vi "提取字符串中数字.vi"(1 "字符串":string) -> (0 "结果":string)   [LabVIEW 2014]
doc: "该模板用于创建子VI。"
panel:
  out "error out":errorcluster caption="错误输出"
  in  "error in (no error)":errorcluster caption="错误输入（无错误）"
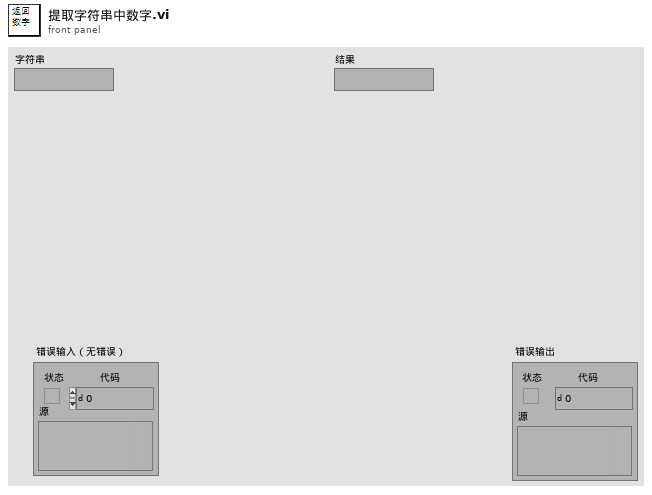
[diagram p1: front panel]
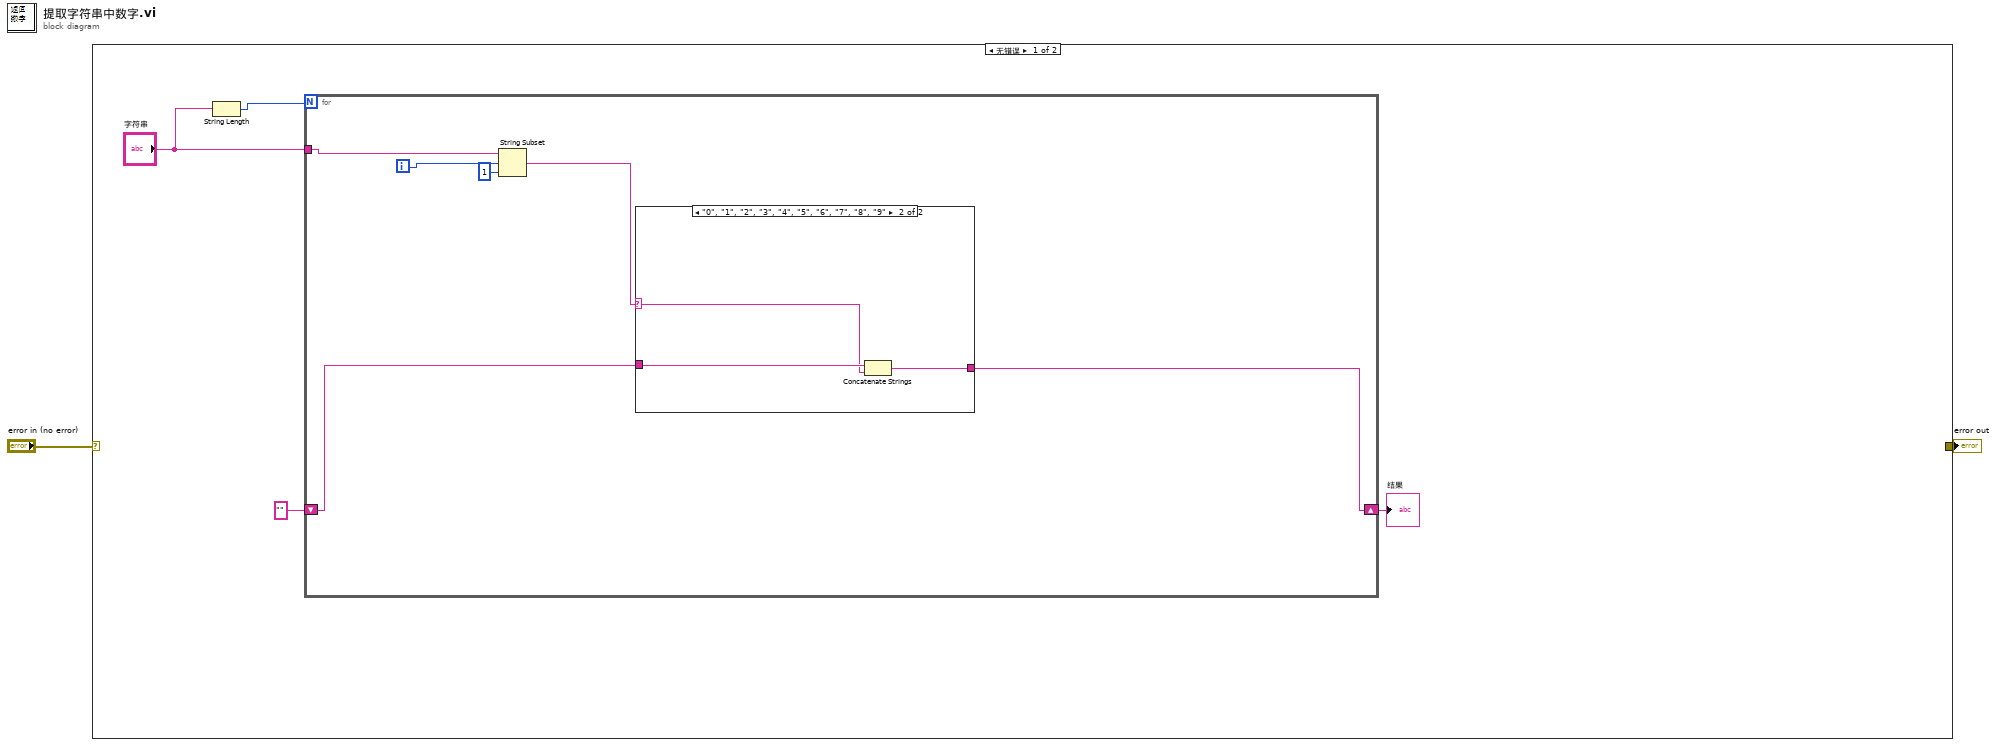
[diagram p0: block diagram]
diagram:
  n1 = case shown="无错误" "error in (no error)" {
    selector: "error in (no error)" -> [_ w17]
    tunnel: [_ w17] -> w1
    frame No Error {
      n2 = String Length(string="字符串") -> (length=w5:i32)
      n3 = for {
        N: w5 -> [_]
        tunnel: "字符串" -> [w12]
        shift-right: [w8] -> w3
        shift-left: "" -> [w9]
        i -> [w11]
        n4 = String Subset(string=w12, offset (0)=w11, length (rest)=1 ("长度（剩余）")) -> (substring=w10:string)
        n5 = case shown="\"0\", \"1\", \"2\", \"3\", \"4\", \"5\", \"6\", \"7\", \"8\", \"9\"" w10 {
          selector: w10 -> [_ w15]
          tunnel: w9 -> [w13 w16]
          tunnel: [w13 w14] -> w8
          frame Default {
          }
          frame "0", "1", "2", "3", "4", "5", "6", "7", "8", "9" {
            n6 = Concatenate Strings(w16, w15) -> (w14:string)
          }
        }
      }
      "结果" <- w3
    }
    frame Error {
    }
  }
  "error out" <- w1
